vi "Create Caption String.vi"(0 "PDF Report IN":refnum<class "PDF Report Class.lvclass">, 2 "Image or Table":T1, 7 "Caption IN":string, 11 "error in (no error)":errorcluster) -> (4 "PDF Report OUT":refnum<class "PDF Report Class.lvclass">, 6 "Font":T2={"Name"="", "Size"=-1.0, "Color"=0, "Style"={"Bold"=FALSE, "Italic"=FALSE, "Underline"=FALSE, "Strikeout"=FALSE}, "Type"={"Type&direction"=enum."Select", "Embedded"=FALSE, "Encoding"=""}}, 8 "Caption OUT":string, 15 "error out":errorcluster)   [LabVIEW 2019, in "Exaprom PDF.lvlib"]
doc: "Version 2.0\nDeveloped by Jean-Marc Simard\nCopyright © 2012, Exaprom Inc.\nAll rights reserved.\nLicense: BSD\n\nWith iTextSharp 4.1.6 (http://itextsharp.sourceforge.net)\nunder Mozilla Public License Version 1.1\n(http://www.mozilla.org/MPL/MPL-1.1.html)"
uses:
  LV Class/PDF Report Class/PDF Report Class.lvclass
  Controls/Font Controls/Font complete cluster.ctl
  Controls/Font Controls/Font size.ctl
  Controls/Font Controls/Font color.ctl
  Controls/Font Controls/Type and encoding.ctl
  Controls/Text Controls/Unicode/Type and run direction.ctl
  Not  in the library/Images for controls/Image or Table.ctl
  Controls/Font Controls/Font complete cluster horizontal.ctl
  Exaprom PDF.lvlib
  LV Class/Fonts Class/Font Class.lvclass
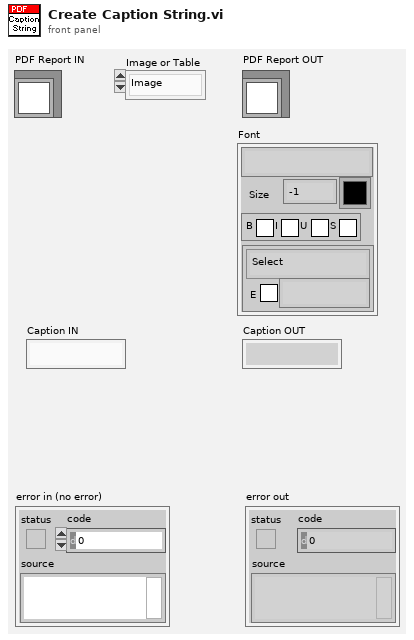
[diagram p1: front panel]
types:
  T1 = typedef "Exaprom PDF.lvlib/Image or Table.ctl" = enum16{"Image", "Table"}
  T2 = typedef "Exaprom PDF.lvlib/Font complete cluster.ctl" = cluster{"Name":string, "Size":T3, "Color":T4, "Style":cluster{"Bold":bool, "Italic":bool, "Underline":bool, "Strikeout":bool}, "Type":T5}
  T3 = typedef "Exaprom PDF.lvlib/Font size.ctl" = sgl
  T4 = typedef "Exaprom PDF.lvlib/Font color.ctl" = u32
  T5 = typedef "Exaprom PDF.lvlib/Type and encoding.ctl" = cluster{"Type&direction":T6, "Embedded":bool, "Encoding":string}
  T6 = typedef "Exaprom PDF.lvlib/Type and run direction.ctl" = enum16{"Select", "ASCII", "UTF-16", "UTF-16 (default)", "UTF-16 (LTR)", "UTF-16 (RTL)"}
  T7 = typedef "Exaprom PDF.lvlib/Font complete cluster horizontal.ctl" = cluster{"Name":string, "Size":T3, "Color":T4, "Style":cluster{"Bold":bool, "Italic":bool, "Underline":bool, "Strikeout":bool}, "Type":T5}
  T8 = typedef "Exaprom PDF.lvlib/Captions.ctl" = cluster{"Figure":T9, "Table":T9, "Font":T2}
  T9 = typedef "Exaprom PDF.lvlib/Image or Table Caption.ctl" = cluster{"Caption":string, "Separator":string, "Position":enum16{"Above", "Below"}}
  T10 = cluster{"Captions":T8, "Image counter":u16, "Table counter":u16}
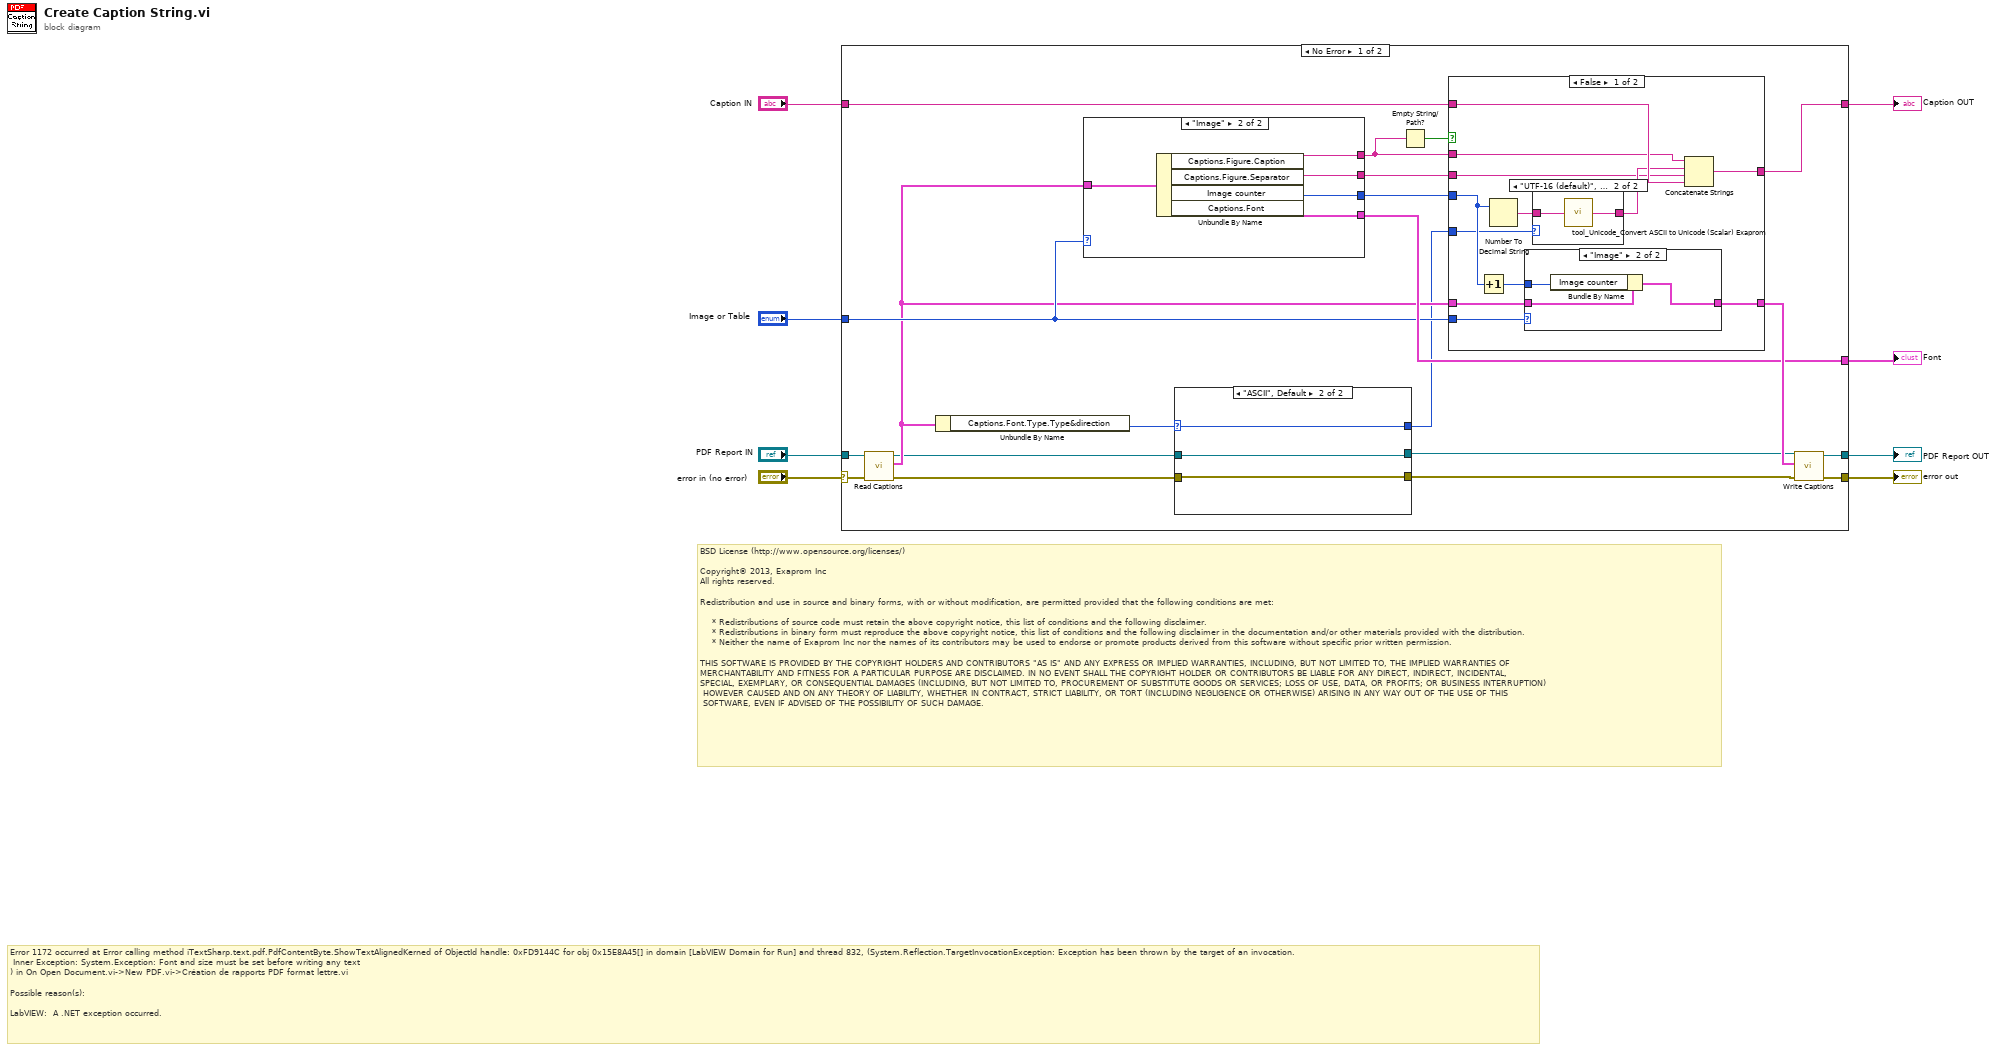
[diagram p0: block diagram]
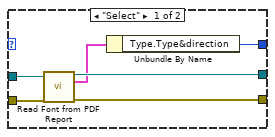
[diagram p2: hidden frame]
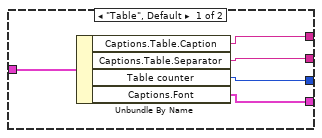
[diagram p3: hidden frame]
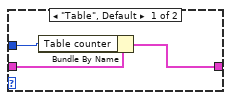
[diagram p4: hidden frame]
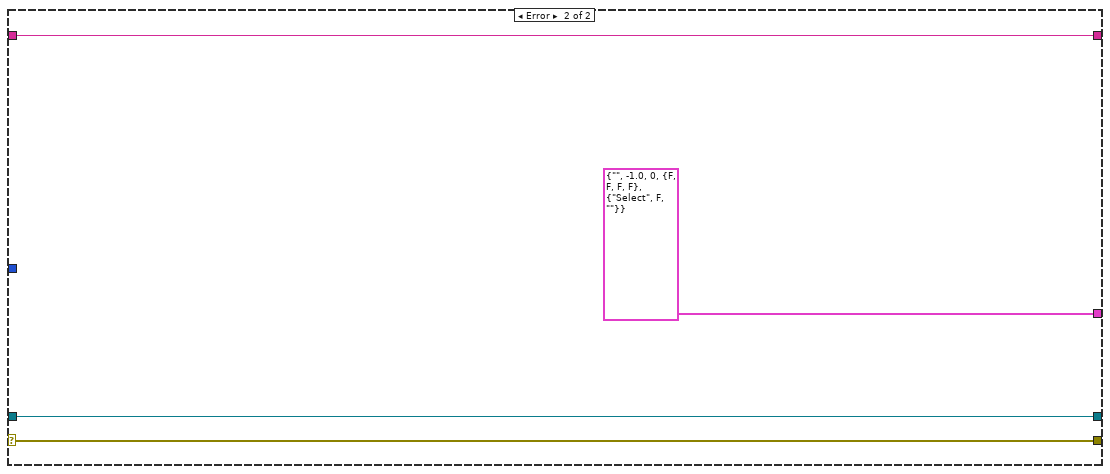
[diagram p7: hidden frame]
diagram:
  # "Error 1172 occurred at Error calling method iTextSharp.text.pdf.PdfContentByte.ShowTextAlignedKerned of ObjectId handle: 0xFD9144C for obj 0x15E8A45[] in domain [LabVIEW Domain for Run] and thread 832, (System.Reflection.TargetInvocationException: Exception has been thrown by the target of an invocation.\n\tInner Exception: System.Exception: Font and size must be set before writing any text\n) in On Open Document.vi->New PDF.vi->Création de rapports PDF format lettre.vi\n\nPossible reason(s):\n\nLabVIEW:  A .NET exception occurred."
  # "BSD License (http://www.opensource.org/licenses/)\n\nCopyright© 2013, Exaprom Inc\nAll rights reserved.\n\nRedistribution and use in source and binary forms, with or without modification, are permitted provided that the following conditions are met:\n\n    * Redistributions of source code must retain the above copyright notice, this list of conditions and the following disclaimer.\n    * Redistributions in binary form must reproduce the above copyright notice, this list of conditions and the following disclaimer in the documentation and/or other materials provided with the distribution.\n    * Neither the name of Exaprom Inc nor the names of its contributors may be used to endorse or promote products derived from this software without specific prior written permission.\n\nTHIS SOFTWARE IS PROVIDED BY THE COPYRIGHT HOLDERS AND CONTRIBUTORS \"AS IS\" AND ANY EXPRESS OR IMPLIED WARRANTIES, INCLUDING, BUT NOT LIMITED TO, THE IMPLIED WARRANTIES OF \nMERCHANTABILITY AND FITNESS FOR A PARTICULAR PURPOSE ARE DISCLAIMED. IN NO EVENT SHALL THE COPYRIGHT HOLDER OR CONTRIBUTORS BE LIABLE FOR ANY DIRECT, INDIRECT, INCIDENTAL,\nSPECIAL, EXEMPLARY, OR CONSEQUENTIAL DAMAGES (INCLUDING, BUT NOT LIMITED TO, PROCUREMENT OF SUBSTITUTE GOODS OR SERVICES; LOSS OF USE, DATA, OR PROFITS; OR BUSINESS INTERRUPTION)\n HOWEVER CAUSED AND ON ANY THEORY OF LIABILITY, WHETHER IN CONTRACT, STRICT LIABILITY, OR TORT (INCLUDING NEGLIGENCE OR OTHERWISE) ARISING IN ANY WAY OUT OF THE USE OF THIS\n SOFTWARE, EVEN IF ADVISED OF THE POSSIBILITY OF SUCH DAMAGE."
  n1 = case shown="No Error" "error in (no error)" {
    selector: "error in (no error)" -> [w24 w74]
    tunnel: "PDF Report IN" -> [w23 w73]
    tunnel: [w18 w73] -> w7
    tunnel: [w19 w74] -> w6
    tunnel: "Caption IN" -> [w22 w72]
    tunnel: [w21 w72] -> w2
    tunnel: [w17 T7 {"Name"="", "Size"=-1.0, "Color"=0, "Style"={"Bold"=FALSE, "Italic"=FALSE, "Underline"=FALSE, "Strikeout"=FALSE}, "Type"={"Type&direction"=enum."Select", "Embedded"=FALSE, "Encoding"=""}} ("Font")] -> w3
    tunnel: "Image or Table" -> [w16 _]
    frame No Error {
      n2 = call-dynamic "Read Captions.vi"("error in (no error)"=w24, "PDF Report Class in"=w23) -> ("error out"=w12:errorcluster, "Captions and counters"=w15:T10, "PDF Report Class out"=w13:refnum<class "PDF Report Class.lvclass">)  [unwired: 7 in]
      n3 = Unbundle By Name(w15) -> ("Captions.Font.Type.Type&direction"=w14:T6)
      n4 = case shown="\"Image\"" w16 {
        tunnel: [w42 w47] -> w28
        tunnel: [w41 w46] -> w27
        tunnel: [w40 w45] -> w26
        tunnel: [w39 w44] -> w17
        tunnel: w15 -> [w38 w43]
        frame "Table", Default {
          n5 = Unbundle By Name(w38) -> ("Captions.Table.Caption"=w40:string, "Captions.Table.Separator"=w41:string, "Table counter"=w42:u16, "Captions.Font"=w39:T2)
        }
        frame "Image" {
          n6 = Unbundle By Name(w43) -> ("Captions.Figure.Caption"=w45:string, "Captions.Figure.Separator"=w46:string, "Image counter"=w47:u16, "Captions.Font"=w44:T2)
        }
      }
      n7 = case shown="\"ASCII\", Default" w14 {
        selector: w14 -> [_ w35]
        tunnel: w13 -> [w34 w37]
        tunnel: w12 -> [w33 w36]
        tunnel: [w32 w37] -> w11
        tunnel: [w31 w36] -> w10
        tunnel: [w29 w35] -> w9
        frame "Select" {
          n8 = call "Read Font from PDF Report.vi"("PDF Report"=w34, "error in (no error)"=w33) -> ("PDF Report duplicate"=w32:refnum<class "PDF Report Class.lvclass">, "Font OUT"=w30:T2, "error out"=w31:errorcluster)  [unwired: 7 in, 4 out]
          n9 = Unbundle By Name(w30) -> ("Type.Type&direction"=w29:T6)
        }
        frame "ASCII", Default {
        }
      }
      n10 = Empty String/Path?(string/path=w26) -> (empty?=w25:bool)
      n11 = case shown="False" w25 {
        tunnel: w22 -> [w58 w70]
        tunnel: w26 -> [w49 _]
        tunnel: w27 -> [w48 _]
        tunnel: w28 -> [w57 _]
        tunnel: [w53 w70] -> w21
        tunnel: w15 -> [w56 w69]
        tunnel: [w54 w69] -> w20
        tunnel: w9 -> [w51 _]
        tunnel: w16 -> [w50 _]
        frame False {
          n12 = Increment(x=w57) -> (x+1=w55:u16)
          n13 = Number To Decimal String(number=w57) -> (decimal integer string=w59:string)  [unwired: 1 out]
          n14 = case shown="\"Image\"" w50 {
            tunnel: w56 -> [w62 w65]
            tunnel: w55 -> [w61 w64]
            tunnel: [w60 w63] -> w54
            frame "Table", Default {
              n15 = Bundle By Name(cluster=w62, "Table counter"=w61) -> (w60:T10)
            }
            frame "Image" {
              n16 = Bundle By Name(cluster=w65, "Image counter"=w64) -> (w63:T10)
            }
          }
          n17 = case shown="\"UTF-16 (default)\", Default" w51 {
            tunnel: w59 -> [w66 w68]
            tunnel: [w66 w67] -> w52
            frame "ASCII" {
            }
            frame "UTF-16 (default)", Default {
              n18 = call "tool_Unicode_Convert ASCII to Unicode (Scalar) Exaprom.vi"("ASCII"=w68) -> ("Unicode"=w67:string)  [unwired: 4 in]
            }
          }
          n19 = Concatenate Strings(w49, w52, w48, w58) -> (w53:string)
        }
        frame True {
        }
      }
      n20 = call-dynamic "Write Captions.vi"("error in (no error)"=w10, "Captions and counters"=w20, "PDF Report Class in"=w11) -> ("error out"=w19:errorcluster, "PDF Report Class out"=w18:refnum<class "PDF Report Class.lvclass">)  [unwired: 7 in]
    }
    frame Error {
    }
  }
  "PDF Report OUT" <- w7
  "error out" <- w6
  "Font" <- w3
  "Caption OUT" <- w2
